vi "DisplayJson.vi"(11 "JSON String In":string="[{\"version\":\"1.0.0\",\"header\":{\"creationDate\":\"2022-06-03T00:00:00\",\"remarks\":\"\",\"serialNumber\":\"98172\",\"productNumber\":\"123021.1804\",\"productType\":\"PAA-9L\",\"pressureType\":2,\"productSeries\":\"9L\",\"compensatedTemperatureRange\":{\"min\":-10.0,\"max\":80.0,\"unit\":4},\"compensatedPressureRange\":{\"min\":0.0,\"max\":0.35,\"unit\":3},\"electricSupply\":{\"magnitude\":1.0,\"unit\":18},\"orderNumber\":9990266,\"orderPosition\":3,\"orderTargetDispatchDate\":\"2022-06-02T00:00:00+00:00\",\"customerName\":\"DemoData Inc.\",\"customerNumber\":12345678,\"customerOrderNumber\":\"Cust-9990266-123\",\"customerReferenceNumber\":\"\",\"customerProductT...") -> ()   [LabVIEW 2017] (continued)
unit\":4},\"error\":{\"magnitude\":-0.10108458,\"unit\":4}}}}}},{\"reference\":\"F_12300_XX_0000098765\",\"environmentTarget\":{\"pressure\":{\"magnitude\":0.11,\"unit\":3},\"temperature\":{\"magnitude\":-10.0,\"unit\":4}},\"environment\":{\"pressure\":{\"magnitude\":0.109992,\"unit\":3},\"temperature\":{\"magnitude\":-10.7286,\"unit\":4},\"supply\":{\"magnitude\":1.0,\"unit\":18}},\"raw\":{\"signal\":{\"magnitude\":24.470345525,\"unit\":22},\"bridgeResistance\":{\"magnitude\":3269.7583636,\"unit\":28}},\"compensated\":{\"mathematicalModels\":{\"MM0123\":{\"pressure\":{\"output\":{\"magnitude\":0.109971,\"unit\":3},\"error\":{\"magnitude\":-0.00613506,\"unit\":7}},\"temperature\":{\"output\":{\"magnitude\":-10.8254,\"unit\":4},\"error\":{\"magnitude\":-0.096812482,\"unit\":4}}}}}},{\"reference\":\"F_12300_XX_0000098765\",\"environmentTarget\":{\"pressure\":{\"magnitude\":0.19,\"unit\":3},\"temperature\":{\"magnitude\":-10.0,\"unit\":4}},\"environment\":{\"pressure\":{\"magnitude\":0.190006,\"unit\":3},\"temperature\":{\"magnitude\":-10.7286,\"unit\":4},\"supply\":{\"magnitude\":1.0,\"unit\":18}},\"raw\":{\"signal\":{\"magnitude\":34.98206966,\"unit\":22},\"bridgeResistance\":{\"magnitude\":3265.8445894,\"unit\":28}},\"compensated\":{\"mathematicalModels\":{\"MM0123\":{\"pressure\":{\"output\":{\"magnitude\":0.190012,\"unit\":3},\"error\":{\"magnitude\":0.0016112092,\"unit\":7}},\"temperature\":{\"output\":{\"magnitude\":-10.8312,\"unit\":4},\"error\":{\"magnitude\":-0.10257656,\"unit\":4}}}}}},{\"reference\":\"F_12300_XX_0000098765\",\"environmentTarget\":{\"pressure\":{\"magnitude\":0.27,\"unit\":3},\"temperature\":{\"magnitude\":-10.0,\"unit\":4}},\"environment\":{\"pressure\":{\"magnitude\":0.269998,\"unit\":3},\"temperature\":{\"magnitude\":-10.7286,\"unit\":4},\"supply\":{\"magnitude\":1.0,\"unit\":18}},\"raw\":{\"signal\":{\"magnitude\":45.449475743,\"unit\":22},\"bridgeResistance\":{\"magnitude\":3262.0921678,\"unit\":28}},\"compensated\":{\"mathematicalModels\":{\"MM0123\":{\"pressure\":{\"output\":{\"magnitude\":0.270017,\"unit\":3},\"error\":{\"magnitude\":0.0055226674,\"unit\":7}},\"temperature\":{\"output\":{\"magnitude\":-10.8273,\"unit\":4},\"error\":{\"magnitude\":-0.098622758,\"unit\":4}}}}}},{\"reference\":\"F_12300_XX_0000098765\",\"environmentTarget\":{\"pressure\":{\"magnitude\":0.35,\"unit\":3},\"temperature\":{\"magnitude\":-10.0,\"unit\":4}},\"environment\":{\"pressure\":{\"magnitude\":0.350009,\"unit\":3},\"temperature\":{\"magnitude\":-10.7286,\"unit\":4},\"supply\":{\"magnitude\":1.0,\"unit\":18}},\"raw\":{\"signal\":{\"magnitude\":55.874377223,\"unit\":22},\"bridgeResistance\":{\"magnitude\":3258.4052741,\"unit\":28}},\"compensated\":{\"mathematicalModels\":{\"MM0123\":{\"pressure\":{\"output\":{\"magnitude\":0.350007,\"unit\":3},\"error\":{\"magnitude\":-0.00057771443,\"unit\":7}},\"temperature\":{\"output\":{\"magnitude\":-10.8286,\"unit\":4},\"error\":{\"magnitude\":-0.099950107,\"unit\":4}}}}}},{\"reference\":\"F_12300_XX_0000098765\",\"environmentTarget\":{\"pressure\":{\"magnitude\":0.03,\"unit\":3},\"temperature\":{\"magnitude\":0.0,\"unit\":4}},\"environment\":{\"pressure\":{\"magnitude\":0.03001,\"unit\":3},\"temperature\":{\"magnitude\":-0.629962,\"unit\":4},\"supply\":{\"magnitude\":1.0,\"unit\":18}},\"raw\":{\"signal\":{\"magnitude\":14.35719489,\"unit\":22},\"bridgeResistance\":{\"magnitude\":3342.4540339,\"unit\":28}},\"compensated\":{\"mathematicalModels\":{\"MM0123\":{\"pressure\":{\"output\":{\"magnitude\":0.0300224,\"unit\":3},\"error\":{\"magnitude\":0.0035324864,\"unit\":7}},\"temperature\":{\"output\":{\"magnitude\":-0.734039,\"unit\":4},\"error\":{\"magnitude\":-0.10407669,\"unit\":4}}}}}},{\"reference\":\"F_12300_XX_0000098765\",\"environmentTarget\":{\"pressure\":{\"magnitude\":0.11,\"unit\":3},\"temperature\":{\"magnitude\":0.0,\"unit\":4}},\"environment\":{\"pressure\":{\"magnitude\":0.110005,\"unit\":3},\"temperature\":{\"magnitude\":-0.629962,\"unit\":4},\"supply\":{\"magnitude\":1.0,\"unit\":18}},\"raw\":{\"signal\":{\"magnitude\":24.865877826,\"unit\":22},\"bridgeResistance\":{\"magnitude\":3338.4734949,\"unit\":28}},\"compensated\":{\"mathematicalModels\":{\"MM0123\":{\"pressure\":{\"output\":{\"magnitude\":0.109982,\"unit\":3},\"error\":{\"magnitude\":-0.0065819783,\"unit\":7}},\"temperature\":{\"output\":{\"magnitude\":-0.740867,\"unit\":4},\"error\":{\"magnitude\":-0.1109055,\"unit\":4}}}}}},{\"reference\":\"F_12300_XX_0000098765\",\"environmentTarget\":{\"pressure\":{\"magnitude\":0.19,\"unit\":3},\"temperature\":{\"magnitude\":0.0,\"unit\":4}},\"environment\":{\"pressure\":{\"magnitude\":0.190002,\"unit\":3},\"temperature\":{\"magnitude\":-0.629962,\"unit\":4},\"supply\":{\"magnitude\":1.0,\"unit\":18}},\"raw\":{\"signal\":{\"magnitude\":35.345777185,\"unit\":22},\"bridgeResistance\":{\"magnitude\":3334.6231034,\"unit\":28}},\"compensated\":{\"mathematicalModels\":{\"MM0123\":{\"pressure\":{\"output\":{\"magnitude\":0.190005,\"unit\":3},\"error\":{\"magnitude\":0.00081559666,\"unit\":7}},\"temperature\":{\"output\":{\"magnitude\":-0.739962,\"unit\":4},\"error\":{\"magnitude\":-0.11000039,\"unit\":4}}}}}},{\"reference\":\"F_12300_XX_0000098765\",\"environmentTarget\":{\"pressure\":{\"magnitude\":0.27,\"unit\":3},\"temperature\":{\"magnitude\":0.0,\"unit\":4}},\"environment\":{\"pressure\":{\"magnitude\":0.269996,\"unit\":3},\"temperature\":{\"magnitude\":-0.629962,\"unit\":4},\"supply\":{\"magnitude\":1.0,\"unit\":18}},\"raw\":{\"signal\":{\"magnitude\":45.785089699,\"unit\":22},\"bridgeResistance\":{\"magnitude\":3330.8335258,\"unit\":28}},\"compensated\":{\"mathematicalModels\":{\"MM0123\":{\"pressure\":{\"output\":{\"magnitude\":0.270005,\"unit\":3},\"error\":{\"magnitude\":0.00269941,\"unit\":7}},\"temperature\":{\"output\":{\"magnitude\":-0.741998,\"unit\":4},\"error\":{\"magnitude\":-0.11203587,\"unit\":4}}}}}},{\"reference\":\"F_12300_XX_0000098765\",\"environmentTarget\":{\"pressure\":{\"magnitude\":0.35,\"unit\":3},\"temperature\":{\"magnitude\":0.0,\"unit\":4}},\"environment\":{\"pressure\":{\"magnitude\":0.350004,\"unit\":3},\"temperature\":{\"magnitude\":-0.629962,\"unit\":4},\"supply\":{\"magnitude\":1.0,\"unit\":18}},\"raw\":{\"signal\":{\"magnitude\":56.183541333,\"unit\":22},\"bridgeResistance\":{\"magnitude\":3327.1077427,\"unit\":28}},\"compensated\":{\"mathematicalModels\":{\"MM0123\":{\"pressure\":{\"output\":{\"magnitude\":0.349982,\"unit\":3},\"error\":{\"magnitude\":-0.006236252,\"unit\":7}},\"temperature\":{\"output\":{\"magnitude\":-0.746851,\"unit\":4},\"error\":{\"magnitude\":-0.1168991,\"unit\":4}}}}}},{\"reference\":\"F_12300_XX_0000098765\",\"environmentTarget\":{\"pressure\":{\"magnitude\":0.03,\"unit\":3},\"temperature\":{\"magnitude\":20.0,\"unit\":4}},\"environment\":{\"pressure\":{\"magnitude\":0.0300054,\"unit\":3},\"temperature\":{\"magnitude\":19.5509,\"unit\":4},\"supply\":{\"magnitude\":1.0,\"unit\":18}},\"raw\":{\"signal\":{\"magnitude\":15.236590331,\"unit\":22},\"bridgeResistance\":{\"magnitude\":3497.1803908,\"unit\":28}},\"compensated\":{\"mathematicalModels\":{\"MM0123\":{\"pressure\":{\"output\":{\"magnitude\":0.030014,\"unit\":3},\"error\":{\"magnitude\":0.0024564587,\"unit\":7}},\"temperature\":{\"output\":{\"magnitude\":19.5482,\"unit\":4},\"error\":{\"magnitude\":-0.0026285351,\"unit\":4}}}}}},{\"reference\":\"F_12300_XX_0000098765\",\"environmentTarget\":{\"pressure\":{\"magnitude\":0.11,\"unit\":3},\"temperature\":{\"magnitude\":20.0,\"unit\":4}},\"environment\":{\"pressure\":{\"magnitude\":0.110001,\"unit\":3},\"temperature\":{\"magnitude\":19.5509,\"unit\":4},\"supply\":{\"magnitude\":1.0,\"unit\":18}},\"raw\":{\"signal\":{\"magnitude\":25.734692204,\"unit\":22},\"bridgeResistance\":{\"magnitude\":3493.2367266,\"unit\":28}},\"compensated\":{\"mathematicalModels\":{\"MM0123\":{\"pressure\":{\"output\":{\"magnitude\":0.109981,\"unit\":3},\"error\":{\"magnitude\":-0.0058181449,\"unit\":7}},\"temperature\":{\"output\":{\"magnitude\":19.5458,\"unit\":4},\"error\":{\"magnitude\":-0.005090711,\"unit\":4}}}}}},{\"reference\":\"F_12300_XX_0000098765\",\"environmentTarget\":{\"pressure\":{\"magnitude\":0.19,\"unit\":3},\"temperature\":{\"magnitude\":20.0,\"unit\":4}},\"environment\":{\"pressure\":{\"magnitude\":0.190008,\"unit\":3},\"temperature\":{\"magnitude\":19.5509,\"unit\":4},\"supply\":{\"magnitude\":1.0,\"unit\":18}},\"raw\":{\"signal\":{\"magnitude\":36.207483064,\"unit\":22},\"bridgeResistance\":{\"magnitude\":3489.3656251,\"unit\":28}},\"compensated\":{\"mathematicalModels\":{\"MM0123\":{\"pressure\":{\"output\":{\"magnitude\":0.19001,\"unit\":3},\"error\":{\"magnitude\":0.00064167096,\"unit\":7}},\"temperature\":{\"output\":{\"magnitude\":19.5443,\"unit\":4},\"error\":{\"magnitude\":-0.0066230307,\"unit\":4}}}}}},{\"reference\":\"F_12300_XX_0000098765\",\"environmentTarget\":{\"pressure\":{\"magnitude\":0.27,\"unit\":3},\"temperature\":{\"magnitude\":20.0,\"unit\":4}},\"environment\":{\"pressure\":{\"magnitude\":0.269992,\"unit\":3},\"temperature\":{\"magnitude\":19.5509,\"unit\":4},\"supply\":{\"magnitude\":1.0,\"unit\":18}},\"raw\":{\"signal\":{\"magnitude\":46.643862109,\"unit\":22},\"bridgeResistance\":{\"magnitude\":3485.5374633,\"unit\":28}},\"compensated\":{\"mathematicalModels\":{\"MM0123\":{\"pressure\":{\"output\":{\"magnitude\":0.27002,\"unit\":3},\"error\":{\"magnitude\":0.007911534,\"unit\":7}},\"temperature\":{\"output\":{\"magnitude\":19.5395,\"unit\":4},\"error\":{\"magnitude\":-0.011376165,\"unit\":4}}}}}},{\"reference\":\"F_12300_XX_0000098765\",\"environmentTarget\":{\"pressure\":{\"magnitude\":0.35,\"unit\":3},\"temperature\":{\"magnitude\":20.0,\"unit\":4}},\"environment\":{\"pressure\":{\"magnitude\":0.35001,\"unit\":3},\"temperature\":{\"magnitude\":19.5509,\"unit\":4},\"supply\":{\"magnitude\":1.0,\"unit\":18}},\"raw\":{\"signal\":{\"magnitude\":57.044716282,\"unit\":22},\"bridgeResistance\":{\"magnitude\":3481.8035535,\"unit\":28}},\"compensated\":{\"mathematicalModels\":{\"MM0123\":{\"pressure\":{\"output\":{\"magnitude\":0.350013,\"unit\":3},\"error\":{\"magnitude\":0.00092508939,\"unit\":7}},\"temperature\":{\"output\":{\"magnitude\":19.5378,\"unit\":4},\"error\":{\"magnitude\":-0.013064621,\"unit\":4}}}}}},{\"reference\":\"F_12300_XX_0000098765\",\"environmentTarget\":{\"pressure\":{\"magnitude\":0.03,\"unit\":3},\"temperature\":{\"magnitude\":40.0,\"unit\":4}},\"environment\":{\"pressure\":{\"magnitude\":0.0300054,\"unit\":3},\"temperature\":{\"magnitude\":39.7284,\"unit\":4},\"supply\":{\"magnitude\":1.0,\"unit\":18}},\"raw\":{\"signal\":{\"magnitude\":16.170043434,\"unit\":22},\"bridgeResistance\":{\"magnitude\":3671.7761859,\"unit\":28}},\"compensated\":{\"mathematicalModels\":{\"MM0123\":{\"pressure\":{\"output\":{\"magnitude\":0.030014,\"unit\":3},\"error\":{\"magnitude\":0.0024675575,\"unit\":7}},\"temperature\":{\"output\":{\"magnitude\":39.7209,\"unit\":4},\"error\":{\"magnitude\":-0.0075103645,\"unit\":4}}}}}},{\"reference\":\"F_12300_XX_0000098765\",\"environmentTarget\":{\"pressure\":{\"magnitude\":0.11,\"unit\":3},\"temperature\":{\"magnitude\":40.0,\"unit\":4}},\"environment\":{\"pressure\":{\"magnitude\":0.109997,\"unit\":3},\"temperature\":{\"magnitude\":39.7284,\"unit\":4},\"supply\":{\"magnitude\":1.0,\"unit\":18}},\"raw\":{\"signal\":{\"magnitude\":26.713979902,\"unit\":22},\"bridgeResistance\":{\"magnitude\":3667.8224123,\"unit\":28}},\"compensated\":{\"mathematicalModels\":{\"MM0123\":{\"pressure\":{\"output\":{\"magnitude\":0.109981,\"unit\":3},\"error\":{\"magnitude\":-0.0046876175,\"unit\":7}},\"temperature\":{\"output\":{\"magnitude\":39.7224,\"unit\":4},\"error\":{\"magnitude\":-0.0059907958,\"unit\":4}}}}}},{\"reference\":\"F_12300_XX_0000098765\",\"environmentTarget\":{\"pressure\":{\"magnitude\":0.19,\"unit\":3},\"temperature\":{\"magnitude\":40.0,\"unit\":4}},\"environment\":{\"pressure\":{\"magnitude\":0.190003,\"unit\":3},\"temperature\":{\"magnitude\":39.7284,\"unit\":4},\"supply\":{\"magnitude\":1.0,\"unit\":18}},\"raw\":{\"signal\":{\"magnitude\":37.234510915,\"unit\":22},\"bridgeResistance\":{\"magnitude\":3663.8592487,\"unit\":28}},\"compensated\":{\"mathematicalModels\":{\"MM0123\":{\"pressure\":{\"output\":{\"magnitude\":0.190002,\"unit\":3},\"error\":{\"magnitude\":-0.00039219625,\"unit\":7}},\"temperature\":{\"output\":{\"magnitude\":39.7159,\"unit\":4},\"error\":{\"magnitude\":-0.012538989,\"unit\":4}}}}}},{\"reference\":\"F_12300_XX_0000098765\",\"environmentTarget\":{\"pressure\":{\"magnitude\":0.27,\"unit\":3},\"temperature\":{\"magnitude\":40.0,\"unit\":4}},\"environment\":{\"pressure\":{\"magnitude\":0.269994,\"unit\":3},\"temperature\":{\"magnitude\":39.7284,\"unit\":4},\"supply\":{\"magnitude\":1.0,\"unit\":18}},\"raw\":{\"signal\":{\"magnitude\":47.723016292,\"unit\":22},\"bridgeResistance\":{\"magnitude\":3660.034404,\"unit\":28}},\"compensated\":{\"mathematicalModels\":{\"MM0123\":{\"pressure\":{\"output\":{\"magnitude\":0.270005,\"unit\":3},\"error\":{\"magnitude\":0.0031922947,\"unit\":7}},\"temperature\":{\"output\":{\"magnitude\":39.7171,\"unit\":4},\"error\":{\"magnitude\":-0.011327982,\"unit\":4}}}}}},{\"reference\":\"F_12300_XX_0000098765\",\"environmentTarget\":{\"pressure\":{\"magnitude\":0.35,\"unit\":3},\"temperature\":{\"magnitude\":40.0,\"unit\":4}},\"environment\":{\"pressure\":{\"magnitude\":0.35,\"unit\":3},\"temperature\":{\"magnitude\":39.7284,\"unit\":4},\"supply\":{\"magnitude\":1.0,\"unit\":18}},\"raw\":{\"signal\":{\"magnitude\":58.177833542,\"unit\":22},\"bridgeResistance\":{\"magnitude\":3656.2531705,\"unit\":28}},\"compensated\":{\"mathematicalModels\":{\"MM0123\":{\"pressure\":{\"output\":{\"magnitude\":0.349982,\"unit\":3},\"error\":{\"magnitude\":-0.0050158997,\"unit\":7}},\"temperature\":{\"output\":{\"magnitude\":39.7156,\"unit\":4},\"error\":{\"magnitude\":-0.012822262,\"unit\":4}}}}}},{\"reference\":\"F_12300_XX_0000098765\",\"environmentTarget\":{\"pressure\":{\"magnitude\":0.03,\"unit\":3},\"temperature\":{\"magnitude\":60.0,\"unit\":4}},\"environment\":{\"pressure\":{\"magnitude\":0.0299896,\"unit\":3},\"temperature\":{\"magnitude\":59.8651,\"unit\":4},\"supply\":{\"magnitude\":1.0,\"unit\":18}},\"raw\":{\"signal\":{\"magnitude\":17.187832335,\"unit\":22},\"bridgeResistance\":{\"magnitude\":3863.2233298,\"unit\":28}},\"compensated\":{\"mathematicalModels\":{\"MM0123\":{\"pressure\":{\"output\":{\"magnitude\":0.0299987,\"unit\":3},\"error\":{\"magnitude\":0.0028717398,\"unit\":7}},\"temperature\":{\"output\":{\"magnitude\":59.9234,\"unit\":4},\"error\":{\"magnitude\":0.058282899,\"unit\":4}}}}}},{\"reference\":\"F_12300_XX_0000098765\",\"environmentTarget\":{\"pressure\":{\"magnitude\":0.11,\"unit\":3},\"temperature\":{\"magnitude\":60.0,\"unit\":4}},\"environment\":{\"pressure\":{\"magnitude\":0.110001,\"unit\":3},\"temperature\":{\"magnitude\":59.8651,\"unit\":4},\"supply\":{\"magnitude\":1.0,\"unit\":18}},\"raw\":{\"signal\":{\"magnitude\":27.814712518,\"unit\":22},\"bridgeResistance\":{\"magnitude\":3859.2205231,\"unit\":28}},\"compensated\":{\"mathematicalModels\":{\"MM0123\":{\"pressure\":{\"output\":{\"magnitude\":0.109979,\"unit\":3},\"error\":{\"magnitude\":-0.0063103794,\"unit\":7}},\"temperature\":{\"output\":{\"magnitude\":59.926,\"unit\":4},\"error\":{\"magnitude\":0.060863769,\"unit\":4}}}}}},{\"reference\":\"F_12300_XX_0000098765\",\"environmentTarget\":{\"pressure\":{\"magnitude\":0.19,\"unit\":3},\"temperature\":{\"magnitude\":60.0,\"unit\":4}},\"environment\":{\"pressure\":{\"magnitude\":0.190004,\"unit\":3},\"temperature\":{\"magnitude\":59.8651,\"unit\":4},\"supply\":{\"magnitude\":1.0,\"unit\":18}},\"raw\":{\"signal\":{\"magnitude\":38.421998929,\"unit\":22},\"bridgeResistance\":{\"magnitude\":3855.2626755,\"unit\":28}},\"compensated\":{\"mathematicalModels\":{\"MM0123\":{\"pressure\":{\"output\":{\"magnitude\":0.190009,\"unit\":3},\"error\":{\"magnitude\":0.0015052422,\"unit\":7}},\"temperature\":{\"output\":{\"magnitude\":59.928,\"unit\":4},\"error\":{\"magnitude\":0.062897084,\"unit\":4}}}}}},{\"reference\":\"F_12300_XX_0000098765\",\"environmentTarget\":{\"pressure\":{\"magnitude\":0.27,\"unit\":3},\"temperature\":{\"magnitude\":60.0,\"unit\":4}},\"environment\":{\"pressure\":{\"magnitude\":0.270009,\"unit\":3},\"temperature\":{\"magnitude\":59.8651,\"unit\":4},\"supply\":{\"magnitude\":1.0,\"unit\":18}},\"raw\":{\"signal\":{\"magnitude\":49.001057362,\"unit\":22},\"bridgeResistance\":{\"magnitude\":3851.3299643,\"unit\":28}},\"compensated\":{\"mathematicalModels\":{\"MM0123\":{\"pressure\":{\"output\":{\"magnitude\":0.270026,\"unit\":3},\"error\":{\"magnitude\":0.0049738773,\"unit\":7}},\"temperature\":{\"output\":{\"magnitude\":59.9271,\"unit\":4},\"error\":{\"magnitude\":0.061931949,\"unit\":4}}}}}},{\"reference\":\"F_12300_XX_0000098765\",\"environmentTarget\":{\"pressure\":{\"magnitude\":0.35,\"unit\":3},\"temperature\":{\"magnitude\":60.0,\"unit\":4}},\"environment\":{\"pressure\":{\"magnitude\":0.349991,\"unit\":3},\"temperature\":{\"magnitude\":59.8651,\"unit\":4},\"supply\":{\"magnitude\":1.0,\"unit\":18}},\"raw\":{\"signal\":{\"magnitude\":59.546601014,\"unit\":22},\"bridgeResistance\":{\"magnitude\":3847.5071402,\"unit\":28}},\"compensated\":{\"mathematicalModels\":{\"MM0123\":{\"pressure\":{\"output\":{\"magnitude\":0.349986,\"unit\":3},\"error\":{\"magnitude\":-0.0013828649,\"unit\":7}},\"temperature\":{\"output\":{\"magnitude\":59.9314,\"unit\":4},\"error\":{\"magnitude\":0.066284127,\"unit\":4}}}}}},{\"reference\":\"F_12300_XX_0000098765\",\"environmentTarget\":{\"pressure\":{\"magnitude\":0.03,\"unit\":3},\"temperature\":{\"magnitude\":80.0,\"unit\":4}},\"environment\":{\"pressure\":{\"magnitude\":0.0300019,\"unit\":3},\"temperature\":{\"magnitude\":79.9513,\"unit\":4},\"supply\":{\"magnitude\":1.0,\"unit\":18}},\"raw\":{\"signal\":{\"magnitude\":18.321153868,\"unit\":22},\"bridgeResistance\":{\"magnitude\":4069.1053966,\"unit\":28}},\"compensated\":{\"mathematicalModels\":{\"MM0123\":{\"pressure\":{\"output\":{\"magnitude\":0.0300144,\"unit\":3},\"error\":{\"magnitude\":0.0035595562,\"unit\":7}},\"temperature\":{\"output\":{\"magnitude\":80.038,\"unit\":4},\"error\":{\"magnitude\":0.086665103,\"unit\":4}}}}}},{\"reference\":\"F_12300_XX_0000098765\",\"environmentTarget\":{\"pressure\":{\"magnitude\":0.11,\"unit\":3},\"temperature\":{\"magnitude\":80.0,\"unit\":4}},\"environment\":{\"pressure\":{\"magnitude\":0.109996,\"unit\":3},\"temperature\":{\"magnitude\":79.9513,\"unit\":4},\"supply\":{\"magnitude\":1.0,\"unit\":18}},\"raw\":{\"signal\":{\"magnitude\":29.052383737,\"unit\":22},\"bridgeResistance\":{\"magnitude\":4065.0423127,\"unit\":28}},\"compensated\":{\"mathematicalModels\":{\"MM0123\":{\"pressure\":{\"output\":{\"magnitude\":0.109968,\"unit\":3},\"error\":{\"magnitude\":-0.0079774118,\"unit\":7}},\"temperature\":{\"output\":{\"magnitude\":80.042,\"unit\":4},\"error\":{\"magnitude\":0.09069531,\"unit\":4}}}}}},{\"reference\":\"F_12300_XX_0000098765\",\"environmentTarget\":{\"pressure\":{\"magnitude\":0.19,\"unit\":3},\"temperature\":{\"magnitude\":80.0,\"unit\":4}},\"environment\":{\"pressure\":{\"magnitude\":0.189995,\"unit\":3},\"temperature\":{\"magnitude\":79.9513,\"unit\":4},\"supply\":{\"magnitude\":1.0,\"unit\":18}},\"raw\":{\"signal\":{\"magnitude\":39.772047806,\"unit\":22},\"bridgeResistance\":{\"magnitude\":4061.0469873,\"unit\":28}},\"compensated\":{\"mathematicalModels\":{\"MM0123\":{\"pressure\":{\"output\":{\"magnitude\":0.189997,\"unit\":3},\"error\":{\"magnitude\":0.00068139861,\"unit\":7}},\"temperature\":{\"output\":{\"magnitude\":80.0489,\"unit\":4},\"error\":{\"magnitude\":0.097427787,\"unit\":4}}}}}},{\"reference\":\"F_12300_XX_0000098765\",\"environmentTarget\":{\"pressure\":{\"magnitude\":0.27,\"unit\":3},\"temperature\":{\"magnitude\":80.0,\"unit\":4}},\"environment\":{\"pressure\":{\"magnitude\":0.270006,\"unit\":3},\"temperature\":{\"magnitude\":79.9513,\"unit\":4},\"supply\":{\"magnitude\":1.0,\"unit\":18}},\"raw\":{\"signal\":{\"magnitude\":50.469946475,\"unit\":22},\"bridgeResistance\":{\"magnitude\":4057.0638106,\"unit\":28}},\"compensated\":{\"mathematicalModels\":{\"MM0123\":{\"pressure\":{\"output\":{\"magnitude\":0.27003,\"unit\":3},\"error\":{\"magnitude\":0.0068981956,\"unit\":7}},\"temperature\":{\"output\":{\"magnitude\":80.0528,\"unit\":4},\"error\":{\"magnitude\":0.10143446,\"unit\":4}}}}}},{\"reference\":\"F_12300_XX_0000098765\",\"environmentTarget\":{\"pressure\":{\"magnitude\":0.35,\"unit\":3},\"temperature\":{\"magnitude\":80.0,\"unit\":4}},\"environment\":{\"pressure\":{\"magnitude\":0.349997,\"unit\":3},\"temperature\":{\"magnitude\":79.9513,\"unit\":4},\"supply\":{\"magnitude\":1.0,\"unit\":18}},\"raw\":{\"signal\":{\"magnitude\":61.135471899,\"unit\":22},\"bridgeResistance\":{\"magnitude\":4053.148397,\"unit\":28}},\"compensated\":{\"mathematicalModels\":{\"MM0123\":{\"pressure\":{\"output\":{\"magnitude\":0.349985,\"unit\":3},\"error\":{\"magnitude\":-0.0034971406,\"unit\":7}},\"temperature\":{\"output\":{\"magnitude\":80.059,\"unit\":4},\"error\":{\"magnitude\":0.10760563,\"unit\":4}}}}}}]},{\"version\":\"1.0.0\",\"header\":{\"creationDate\":\"2022-06-03T00:00:00\",\"remarks\":\"\",\"serialNumber\":\"98142\",\"productNumber\":\"123021.1804\",\"productType\":\"PAA-9L\",\"pressureType\":2,\"productSeries\":\"9L\",\"compensatedTemperatureRange\":{\"min\":-10.0,\"max\":80.0,\"unit\":4},\"compensatedPressureRange\":{\"min\":0.0,\"max\":0.35,\"unit\":3},\"electricSupply\":{\"magnitude\":1.0,\"unit\":18},\"orderNumber\":9990266,\"orderPosition\":3,\"orderTargetDispatchDate\":\"2022-06-02T00:00:00+00:00\",\"customerName\":\"DemoData Inc.\",\"customerNumber\":12345678,\"customerOrderNumber\":\"Cust-9990266-123\",\"customerReferenceNumber\":\"\",\"customerProductType\":\"123021-1804 Rev.AA\"},\"compensationMethods\":{\"mathematicalModels\":{\"MM0123\":{\"modelType\":\"MM0123\",\"productNumber\":\"000000.0000\",\"compensatedTemperatureRange\":{\"min\":-10.0,\"max\":80.0,\"unit\":4},\"compensatedPressureRange\":{\"min\":0.0,\"max\":0.35,\"unit\":3},\"electricSupply\":{\"magnitude\":1.0,\"unit\":18},\"parts\":{\"pressure\":{\"inputs\":[\"Sig\",\"R\"],\"output\":\"P\",\"description\":\"P = f(Sig,R)\",\"coefficients\":[[4.29779907342,-0.00434478902614,1.62864479395E-06,-2.73354938748E-10,1.71864034763E-14],[-0.136835659348,0.000146053801046,-5.52910357556E-08,9.29935498533E-12,-5.87609489244E-16],[-0.000204460783497,2.48959743385E-07,-1.10098733855E-10,2.12452900426E-14,-1.51897723151E-18]]},\"temperature\":{\"inputs\":[\"R\",\"Sig\"],\"output\":\"T\",\"description\":\"T = f(R,Sig)\",\"coefficients\":[[-8139.58148913,7.90134196848,-0.0779966126175],[7.95461195444,-0.00741120435127,8.19850589853E-05],[-0.00297948964638,2.60928720307E-06,-3.23355118182E-08],[5.05318369448E-07,-4.0561890458E-10,5.66723534531E-12],[-3.23330043842E-11,2.34055663306E-14,-3.72255851896E-16]]}}}}},\"measurements\":[{\"reference\":\"F_12300_XX_0000098765\",\"environmentTarget\":{\"pressure\":{\"magnitude\":0.03,\"unit\":3},\"temperature\":{\"magnitude\":-10.0,\"unit\":4}},\"environment\":{\"pressure\":{\"magnitude\":0.0299821,\"unit\":3},\"temperature\":{\"magnitude\":-10.7286,\"unit\":4},\"supply\":{\"magnitude\":1.0,\"unit\":18}},\"raw\":{\"signal\":{\"magnitude\":15.776956636,\"unit\":22},\"bridgeResistance\":{\"magnitude\":3293.7496367,\"unit\":28}},\"compensated\":{\"mathematicalModels\":{\"MM0123\":{\"pressure\":{\"output\":{\"magnitude\":0.0299928,\"unit\":3},\"error\":{\"magnitude\":0.0030441522,\"unit\":7}},\"temperature\":{\"output\":{\"magnitude\":-10.8332,\"unit\":4},\"error\":{\"magnitude\":-0.10455635,\"unit\":4}}}}}},{\"reference\":\"F_12300_XX_0000098765\",\"environmentTarget\":{\"pressure\":{\"magnitude\":0.11,\"unit\":3},\"temperature\":{\"magnitude\":-10.0,\"unit\":4}},\"environment\":{\"pressure\":{\"magnitude\":0.109993,\"unit\":3},\"temperature\":{\"magnitude\":-10.7286,\"unit\":4},\"supply\":{\"magnitude\":1.0,\"unit\":18}},\"raw\":{\"signal\":{\"magnitude\":26.294106914,\"unit\":22},\"bridgeResistance\":{\"magnitude\":3289.8095518,\"unit\":28}},\"compensated\":{\"mathematicalModels\":{\"MM0123\":{\"pressure\":{\"output\":{\"magnitude\":0.109968,\"unit\":3},\"error\":{\"magnitude\":-0.0072274761,\"unit\":7}},\"temperature\":{\"output\":{\"magnitude\":-10.8308,\"unit\":4},\"error\":{\"magnitude\":-0.10213503,\"unit\":4}}}}}},{\"reference\":\"F_12300_XX_0000098765\",\"environmentTarget\":{\"pressure\":{\"magnitude\":0.19,\"unit\":3},\"temperature\":{\"magnitude\":-10.0,\"unit\":4}},\"environment\":{\"pressure\":{\"magnitude\":0.190004,\"unit\":3},\"temperature\":{\"magnitude\":-10.7286,\"unit\":4},\"supply\":{\"magnitude\":1.0,\"unit\":18}},\"raw\":{\"signal\":{\"magnitude\":36.781681087,\"unit\":22},\"bridgeResistance\":{\"magnitude\":3285.9207285,\"unit\":28}},\"compensated\":{\"mathematicalModels\":{\"MM0123\":{\"pressure\":{\"output\":{\"magnitude\":0.190014,\"unit\":3},\"error\":{\"magnitude\":0.002929267,\"unit\":7}},\"temperature\":{\"output\":{\"magnitude\":-10.8338,\"unit\":4},\"error\":{\"magnitude\":-0.10512799,\"unit\":4}}}}}},{\"reference\":\"F_12300_XX_0000098765\",\"environmentTarget\":{\"pressure\":{\"magnitude\":0.27,\"unit\":3},\"temperature\":{\"magnitude\":-10.0,\"unit\":4}},\"environment\":{\"pressure\":{\"magnitude\":0.270005,\"unit\":3},\"temperature\":{\"magnitude\":-10.7286,\"unit\":4},\"supply\":{\"magnitude\":1.0,\"unit\":18}},\"raw\":{\"signal\":{\"magnitude\":47.225319124,\"unit\":22},\"bridgeResistance\":{\"magnitude\":3282.1674533,\"unit\":28}},\"compensated\":{\"mathematicalModels\":{\"MM0123\":{\"pressure\":{\"output\":{\"magnitude\":0.270021,\"unit\":3},\"error\":{\"magnitude\":0.0045124949,\"unit\":7}},\"temperature\":{\"output\":{\"magnitude\":-10.8306,\"unit\":4},\"error\":{\"magnitude\":-0.10200542,\"unit\":4}}}}}},{\"reference\":\"F_12300_XX_0000098765\",\"environmentTarget\":{\"pressure\":{\"magnitude\":0.35,\"unit\":3},\"temperature\":{\"magnitude\":-10.0,\"unit\":4}},\"environment\":{\"pressure\":{\"magnitude\":0.350005,\"unit\":3},\"temperature\":{\"magnitude\":-10.7286,\"unit\":4},\"supply\":{\"magnitude\":1.0,\"unit\":18}},\"raw\":{\"signal\":{\"magnitude\":57.626446818,\"unit\":22},\"bridgeResistance\":{\"magnitude\":3278.4696744,\"unit\":28}},\"compensated\":{\"mathematicalModels\":{\"MM0123\":{\"pressure\":{\"output\":{\"magnitude\":0.350002,\"unit\":3},\"error\":{\"magnitude\":-0.00086307966,\"unit\":7}},\"temperature\":{\"output\":{\"magnitude\":-10.8338,\"unit\":4},\"error\":{\"magnitude\":-0.10512444,\"unit\":4}}}}}},{\"reference\":\"F_12300_XX_0000098765\",\"environmentTarget\":{\"pressure\":{\"magnitude\":0.03,\"unit\":3},\"temperature\":{\"magnitude\":0.0,\"unit\":4}},\"environment\":{\"pressure\":{\"magnitude\":0.0300035,\"unit\":3},\"temperature\":{\"magnitude\":-0.629962,\"unit\":4},\"supply\":{\"magnitude\":1.0,\"unit\":18}},\"raw\":{\"signal\":{\"magnitude\":16.216359492,\"unit\":22},\"bridgeResistance\":{\"magnitude\":3363.1917989,\"unit\":28}},\"compensated\":{\"mathematicalModels\":{\"MM0123\":{\"pressure\":{\"output\":{\"magnitude\":0.0300209,\"unit\":3},\"error\":{\"magnitude\":0.0049814934,\"unit\":7}},\"temperature\":{\"output\":{\"magnitude\":-0.737174,\"unit\":4},\"error\":{\"magnitude\":-0.10721222,\"unit\":4}}}}}},{\"reference\":\"F_12300_XX_0000098765\",\"environmentTarget\":{\"pressure\":{\"magnitude\":0.11,\"unit\":3},\"temperature\":{\"magnitude\":0.0,\"unit\":4}},\"environment\":{\"pressure\":{\"magnitude\":0.110002,\"unit\":3},\"temperature\":{\"magnitude\":-0.629962,\"unit\":4},\"supply\":{\"magnitude\":1.0,\"unit\":18}},\"raw\":{\"signal\":{\"magnitude\":26.700152723,\"unit\":22},\"bridgeResistance\":{\"magnitude\":3359.2162873,\"unit\":28}},\"compensated\":{\"mathematicalModels\":{\"MM0123\":{\"pressure\":{\"output\":{\"magnitude\":0.109979,\"unit\":3},\"error\":{\"magnitude\":-0.0065580569,\"unit\":7}},\"temperature\":{\"output\":{\"magnitude\":-0.743391,\"unit\":4},\"error\":{\"magnitude\":-0.11342921,\"unit\":4}}}}}},{\"reference\":\"F_12300_XX_0000098765\",\"environmentTarget\":{\"pressure\":{\"magnitude\":0.19,\"unit\":3},\"temperature\":{\"magnitude\":0.0,\"unit\":4}},\"environment\":{\"pressure\":{\"magnitude\":0.190003,\"unit\":3},\"temperature\":{\"magnitude\":-0.629962,\"unit\":4},\"supply\":{\"magnitude\":1.0,\"unit\":18}},\"raw\":{\"signal\":{\"magnitude\":37.15630133,\"unit\":22},\"bridgeResistance\":{\"magnitude\":3355.3509745,\"unit\":28}},\"compensated\":{\"mathematicalModels\":{\"MM0123\":{\"pressure\":{\"output\":{\"magnitude\":0.190006,\"unit\":3},\"error\":{\"magnitude\":0.00083240384,\"unit\":7}},\"temperature\":{\"output\":{\"magnitude\":-0.744849,\"unit\":4},\"error\":{\"magnitude\":-0.11489762,\"unit\":4}}}}}},{\"reference\":\"F_12300_XX_0000098765\",\"environmentTarget\":{\"pressure\":{\"magnitude\":0.27,\"unit\":3},\"temperature\":{\"magnitude\":0.0,\"unit\":4}},\"environment\":{\"pressure\":{\"magnitude\":0.269996,\"unit\":3},\"temperature\":{\"magnitude\":-0.629962,\"unit\":4},\"supply\":{\"magnitude\":1.0,\"unit\":18}},\"raw\":{\"signal\":{\"magnitude\":47.572349784,\"unit\":22},\"bridgeResistance\":{\"magnitude\":3351.5811672,\"unit\":28}},\"compensated\":{\"mathematicalModels\":{\"MM0123\":{\"pressure\":{\"output\":{\"magnitude\":0.270008,\"unit\":3},\"error\":{\"magnitude\":0.0034977634,\"unit\":7}},\"temperature\":{\"output\":{\"magnitude\":-0.744483,\"unit\":4},\"error\":{\"magnitude\":-0.11452151,\"unit\":4}}}}}},{\"reference\":\"F_12300_XX_0000098765\",\"environmentTarget\":{\"pressure\":{\"magnitude\":0.35,\"unit\":3},\"temperature\":{\"magnitude\":0.0,\"unit\":4}},\"environment\":{\"pressure\":{\"magnitude\":0.350001,\"unit\":3},\"temperature\":{\"magnitude\":-0.629962,\"unit\":4},\"supply\":{\"magnitude\":1.0,\"unit\":18}},\"raw\":{\"signal\":{\"magnitude\":57.947679068,\"unit\":22},\"bridgeResistance\":{\"magnitude\":3347.8649258,\"unit\":28}},\"compensated\":{\"mathematicalModels\":{\"MM0123\":{\"pressure\":{\"output\":{\"magnitude\":0.349983,\"unit\":3},\"error\":{\"magnitude\":-0.0050333892,\"unit\":7}},\"temperature\":{\"output\":{\"magnitude\":-0.748403,\"unit\":4},\"error\":{\"magnitude\":-0.11844154,\"unit\":4}}}}}},{\"reference\":\"F_12300_XX_0000098765\",\"environmentTarget\":{\"pressure\":{\"magnitude\":0.03,\"unit\":3},\"temperature\":{\"magnitude\":20.0,\"unit\":4}},\"environment\":{\"pressure\":{\"magnitude\":0.0300021,\"unit\":3},\"temperature\":{\"magnitude\":19.5509,\"unit\":4},\"supply\":{\"magnitude\":1.0,\"unit\":18}},\"raw\":{\"signal\":{\"magnitude\":17.125518981,\"unit\":22},\"bridgeResistance\":{\"magnitude\":3519.3757607,\"unit\":28}},\"compensated\":{\"mathematicalModels\":{\"MM0123\":{\"pressure\":{\"output\":{\"magnitude\":0.0300077,\"unit\":3},\"error\":{\"magnitude\":0.0016139562,\"unit\":7}},\"temperature\":{\"output\":{\"magnitude\":19.5458,\"unit\":4},\"error\":{\"magnitude\":-0.0051155368,\"unit\":4}}}}}},{\"reference\":\"F_12300_XX_0000098765\",\"environmentTarget\":{\"pressure\":{\"magnitude\":0.11,\"unit\":3},\"temperature\":{\"magnitude\":20.0,\"unit\":4}},\"environment\":{\"pressure\":{\"magnitude\":0.109997,\"unit\":3},\"temperature\":{\"magnitude\":19.5509,\"unit\":4},\"supply\":{\"magnitude\":1.0,\"unit\":18}},\"raw\":{\"signal\":{\"magnitude\":27.598966245,\"unit\":22},\"bridgeResistance\":{\"magnitude\":3515.4423761,\"unit\":28}},\"compensated\":{\"mathematicalModels\":{\"MM0123\":{\"pressure\":{\"output\":{\"magnitude\":0.109971,\"unit\":3},\"error\":{\"magnitude\":-0.0072892523,\"unit\":7}},\"temperature\":{\"output\":{\"magnitude\":19.5444,\"unit\":4},\"error\":{\"magnitude\":-0.0064308564,\"unit\":4}}}}}},{\"reference\":\"F_12300_XX_0000098765\",\"environmentTarget\":{\"pressure\":{\"magnitude\":0.19,\"unit\":3},\"temperature\":{\"magnitude\":20.0,\"unit\":4}},\"environment\":{\"pressure\":{\"magnitude\":0.189997,\"unit\":3},\"temperature\":{\"magnitude\":19.5509,\"unit\":4},\"supply\":{\"magnitude\":1.0,\"unit\":18}},\"raw\":{\"signal\":{\"magnitude\":38.048487108,\"unit\":22},\"bridgeResistance\":{\"magnitude\":3511.5684274,\"unit\":28}},\"compensated\":{\"mathematicalModels\":{\"MM0123\":{\"pressure\":{\"output\":{\"magnitude\":0.190004,\"unit\":3},\"error\":{\"magnitude\":0.0018700724,\"unit\":7}},\"temperature\":{\"output\":{\"magnitude\":19.5425,\"unit\":4},\"error\":{\"magnitude\":-0.0084008002,\"unit\":4}}}}}},{\"reference\":\"F_12300_XX_0000098765\",\"environmentTarget\":{\"pressure\":{\"magnitude\":0.27,\"unit\":3},\"temperature\":{\"magnitude\":20.0,\"unit\":4}},\"environment\":{\"pressure\":{\"magnitude\":0.269993,\"unit\":3},\"temperature\":{\"magnitude\":19.5509,\"unit\":4},\"supply\":{\"magnitude\":1.0,\"unit\":18}},\"raw\":{\"signal\":{\"magnitude\":48.462584839,\"unit\":22},\"bridgeResistance\":{\"magnitude\":3507.7445967,\"unit\":28}},\"compensated\":{\"mathematicalModels\":{\"MM0123\":{\"pressure\":{\"output\":{\"magnitude\":0.270017,\"unit\":3},\"error\":{\"magnitude\":0.0068983906,\"unit\":7}},\"temperature\":{\"output\":{\"magnitude\":19.5382,\"unit\":4},\"error\":{\"magnitude\":-0.012725299,\"unit\":4}}}}}},{\"reference\":\"F_12300_XX_0000098765\",\"environmentTarget\":{\"pressure\":{\"magnitude\":0.35,\"unit\":3},\"temperature\":{\"magnitude\":20.0,\"unit\":4}},\"environment\":{\"pressure\":{\"magnitude\":0.350007,\"unit\":3},\"temperature\":{\"magnitude\":19.5509,\"unit\":4},\"supply\":{\"magnitude\":1.0,\"unit\":18}},\"raw\":{\"signal\":{\"magnitude\":58.8404609,\"unit\":22},\"bridgeResistance\":{\"magnitude\":3503.9948594,\"unit\":28}},\"compensated\":{\"mathematicalModels\":{\"MM0123\":{\"pressure\":{\"output\":{\"magnitude\":0.350005,\"unit\":3},\"error\":{\"magnitude\":-0.00055217311,\"unit\":7}},\"temperature\":{\"output\":{\"magnitude\":19.5343,\"unit\":4},\"error\":{\"magnitude\":-0.016584369,\"unit\":4}}}}}},{\"reference\":\"F_12300_XX_0000098765\",\"environmentTarget\":{\"pressure\":{\"magnitude\":0.03,\"unit\":3},\"temperature\":{\"magnitude\":40.0,\"unit\":4}},\"environment\":{\"pressure\":{\"magnitude\":0.0299921,\"unit\":3},\"temperature\":{\"magnitude\":39.7284,\"unit\":4},\"supply\":{\"magnitude\":1.0,\"unit\":18}},\"raw\":{\"signal\":{\"magnitude\":18.103510464,\"unit\":22},\"bridgeResistance\":{\"magnitude\":3695.5684626,\"unit\":28}},\"compensated\":{\"mathematicalModels\":{\"MM0123\":{\"pressure\":{\"output\":{\"magnitude\":0.030005,\"unit\":3},\"error\":{\"magnitude\":0.0036854103,\"unit\":7}},\"temperature\":{\"output\":{\"magnitude\":39.7216,\"unit\":4},\"error\":{\"magnitude\":-0.0068102955,\"unit\":4}}}}}},{\"reference\":\"F_12300_XX_0000098765\",\"environmentTarget\":{\"pressure\":{\"magnitude\":0.11,\"unit\":3},\"temperature\":{\"magnitude\":40.0,\"unit\":4}},\"environment\":{\"pressure\":{\"magnitude\":0.109997,\"unit\":3},\"temperature\":{\"magnitude\":39.7284,\"unit\":4},\"supply\":{\"magnitude\":1.0,\"unit\":18}},\"raw\":{\"signal\":{\"magnitude\":28.623694468,\"unit\":22},\"bridgeResistance\":{\"magnitude\":3691.6051995,\"unit\":28}},\"compensated\":{\"mathematicalModels\":{\"MM0123\":{\"pressure\":{\"output\":{\"magnitude\":0.109977,\"unit\":3},\"error\":{\"magnitude\":-0.0056026922,\"unit\":7}},\"temperature\":{\"output\":{\"magnitude\":39.7212,\"unit\":4},\"error\":{\"magnitude\":-0.0071787919,\"unit\":4}}}}}},{\"reference\":\"F_12300_XX_0000098765\",\"environmentTarget\":{\"pressure\":{\"magnitude\":0.19,\"unit\":3},\"temperature\":{\"magnitude\":40.0,\"unit\":4}},\"environment\":{\"pressure\":{\"magnitude\":0.190002,\"unit\":3},\"temperature\":{\"magnitude\":39.7284,\"unit\":4},\"supply\":{\"magnitude\":1.0,\"unit\":18}},\"raw\":{\"signal\":{\"magnitude\":39.121526401,\"unit\":22},\"bridgeResistance\":{\"magnitude\":3687.6533329,\"unit\":28}},\"compensated\":{\"mathematicalModels\":{\"MM0123\":{\"pressure\":{\"output\":{\"magnitude\":0.190003,\"unit\":3},\"error\":{\"magnitude\":0.00019345344,\"unit\":7}},\"temperature\":{\"output\":{\"magnitude\":39.7153,\"unit\":4},\"error\":{\"magnitude\":-0.01310946,\"unit\":4}}}}}},{\"reference\":\"F_12300_XX_0000098765\",\"environmentTarget\":{\"pressure\":{\"magnitude\":0.27,\"unit\":3},\"temperature\":{\"magnitude\":40.0,\"unit\":4}},\"environment\":{\"pressure\":{\"magnitude\":0.269996,\"unit\":3},\"temperature\":{\"magnitude\":39.7284,\"unit\":4},\"supply\":{\"magnitude\":1.0,\"unit\":18}},\"raw\":{\"signal\":{\"magnitude\":49.58946532,\"unit\":22},\"bridgeResistance\":{\"magnitude\":3683.8470407,\"unit\":28}},\"compensated\":{\"mathematicalModels\":{\"MM0123\":{\"pressure\":{\"output\":{\"magnitude\":0.27001,\"unit\":3},\"error\":{\"magnitude\":0.0039132686,\"unit\":7}},\"temperature\":{\"output\":{\"magnitude\":39.718,\"unit\":4},\"error\":{\"magnitude\":-0.0103763,\"unit\":4}}}}}},{\"reference\":\"F_12300_XX_0000098765\",\"environmentTarget\":{\"pressure\":{\"magnitude\":0.35,\"unit\":3},\"temperature\":{\"magnitude\":40.0,\"unit\":4}},\"environment\":{\"pressure\":{\"magnitude\":0.349999,\"unit\":3},\"temperature\":{\"magnitude\":39.7284,\"unit\":4},\"supply\":{\"magnitude\":1.0,\"unit\":18}},\"raw\":{\"signal\":{\"magnitude\":60.021983002,\"unit\":22},\"bridgeResistance\":{\"magnitude\":3680.0673502,\"unit\":28}},\"compensated\":{\"mathematicalModels\":{\"MM0123\":{\"pressure\":{\"output\":{\"magnitude\":0.349985,\"unit\":3},\"error\":{\"magnitude\":-0.0041199458,\"unit\":7}},\"temperature\":{\"output\":{\"magnitude\":39.7164,\"unit\":4},\"error\":{\"magnitude\":-0.012016896,\"unit\":4}}}}}},{\"reference\":\"F_12300_XX_0000098765\",\"environmentTarget\":{\"pressure\":{\"magnitude\":0.03,\"unit\":3},\"temperature\":{\"magnitude\":60.0,\"unit\":4}},\"environment\":{\"pressure\":{\"magnitude\":0.0299913,\"unit\":3},\"temperature\":{\"magnitude\":59.8651,\"unit\":4},\"supply\":{\"magnitude\":1.0,\"unit\":18}},\"raw\":{\"signal\":{\"magnitude\":19.183641173,\"unit\":22},\"bridgeResistance\":{\"magnitude\":3898.7414528,\"unit\":28}},\"compensated\":{\"mathematicalModels\":{\"MM0123\":{\"pressure\":{\"output\":{\"magnitude\":0.0300014,\"unit\":3},\"error\":{\"magnitude\":0.0028935226,\"unit\":7}},\"temperature\":{\"output\":{\"magnitude\":59.9254,\"unit\":4},\"error\":{\"magnitude\":0.06030113,\"unit\":4}}}}}},{\"reference\":\"F_12300_XX_0000098765\",\"environmentTarget\":{\"pressure\":{\"magnitude\":0.11,\"unit\":3},\"temperature\":{\"magnitude\":60.0,\"unit\":4}},\"environment\":{\"pressure\":{\"magnitude\":0.109997,\"unit\":3},\"temperature\":{\"magnitude\":59.8651,\"unit\":4},\"supply\":{\"magnitude\":1.0,\"unit\":18}},\"raw\":{\"signal\":{\"magnitude\":29.785943165,\"unit\":22},\"bridgeResistance\":{\"magnitude\":3894.73899,\"unit\":28}},\"compensated\":{\"mathematicalModels\":{\"MM0123\":{\"pressure\":{\"output\":{\"magnitude\":0.109973,\"unit\":3},\"error\":{\"magnitude\":-0.0067300332,\"unit\":7}},\"temperature\":{\"output\":{\"magnitude\":59.9276,\"unit\":4},\"error\":{\"magnitude\":0.062434406,\"unit\":4}}}}}},{\"reference\":\"F_12300_XX_0000098765\",\"environmentTarget\":{\"pressure\":{\"magnitude\":0.19,\"unit\":3},\"temperature\":{\"magnitude\":60.0,\"unit\":4}},\"environment\":{\"pressure\":{\"magnitude\":0.190003,\"unit\":3},\"temperature\":{\"magnitude\":59.8651,\"unit\":4},\"supply\":{\"magnitude\":1.0,\"unit\":18}},\"raw\":{\"signal\":{\"magnitude\":40.371294679,\"unit\":22},\"bridgeResistance\":{\"magnitude\":3890.7926507,\"unit\":28}},\"compensated\":{\"mathematicalModels\":{\"MM0123\":{\"pressure\":{\"output\":{\"magnitude\":0.19001,\"unit\":3},\"error\":{\"magnitude\":0.0020395849,\"unit\":7}},\"temperature\":{\"output\":{\"magnitude\":59.9299,\"unit\":4},\"error\":{\"magnitude\":0.064783614,\"unit\":4}}}}}},{\"reference\":\"F_12300_XX_0000098765\",\"environmentTarget\":{\"pressure\":{\"magnitude\":0.27,\"unit\":3},\"temperature\":{\"magnitude\":60.0,\"unit\":4}},\"environment\":{\"pressure\":{\"magnitude\":0.270008,\"unit\":3},\"temperature\":{\"magnitude\":59.8651,\"unit\":4},\"supply\":{\"magnitude\":1.0,\"unit\":18}},\"
